vi "Data Conversion - Byte Array to Signed 32 Bit Array.vi"(9 "Unsigned Byte Array":u8[](array[numeric]), 10 "Byte Order":T1(ring)) -> (2 "(Signed) 32 Bit Array":i32[](array[numeric]))   [LabVIEW 2017, in "Communications Library.lvlib"]
doc: "Converts a byte array into an array of 32 bit integers"
uses:
  Communications Library.lvlib
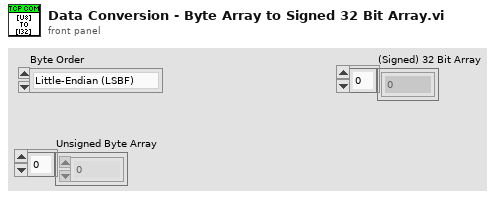
[diagram p1: front panel]
types:
  T1 = enum16{"Little-Endian (LSBF)", "Big-Endian (MSBF)"}
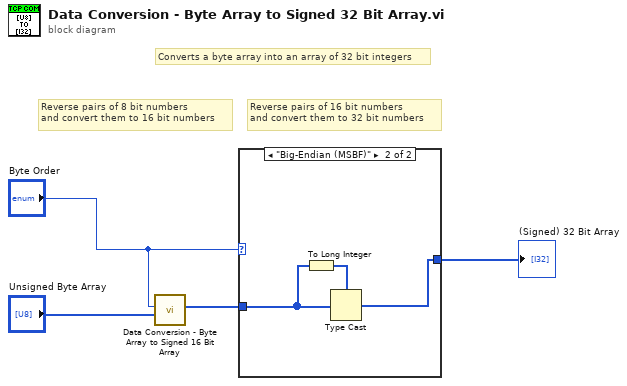
[diagram p0: block diagram]
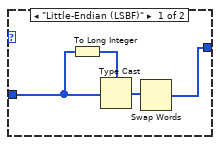
[diagram p2: hidden frame]
diagram:
  # "Reverse pairs of 16 bit numbers\nand convert them to 32 bit numbers"
  # "Reverse pairs of 8 bit numbers\nand convert them to 16 bit numbers"
  # "Converts a byte array into an array of 32 bit integers"
  n1 = call "Data Conversion - Byte Array to Signed 16 Bit Array.vi"("Unsigned Byte Array"="Unsigned Byte Array", "Byte Order"="Byte Order") -> ("(Signed) 16 Bit Array"=w1:i16[])  [unwired: 9 in]
  n2 = case shown="\"Big-Endian (MSBF)\"" "Byte Order" {
    tunnel: w1 -> [w6 w10]
    tunnel: [w7 w11] -> w4
    frame "Little-Endian (LSBF)" {
      n3 = To Long Integer(number=w6) -> (32bit integer=w5:i32[])
      n4 = Type Cast(type=w5, x=w6) -> (*(type *) &x=w8:i32[])
      n5 = Swap Words(1:w8) -> (0:w7:i32[])
    }
    frame "Big-Endian (MSBF)" {
      n6 = To Long Integer(number=w10) -> (32bit integer=w9:i32[])
      n7 = Type Cast(type=w9, x=w10) -> (*(type *) &x=w11:i32[])
    }
  }
  "(Signed) 32 Bit Array" <- w4
